vi "apply_deadband.vi"(10 "Deadband":dbl, 11 "Input":dbl) -> (3 "Input with deadband":dbl)   [LabVIEW 2012]
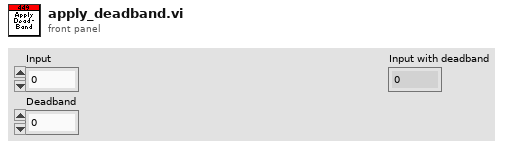
[diagram p1: front panel]
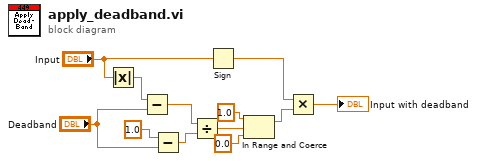
[diagram p0: block diagram]
diagram:
  n1 = Absolute Value(x="Input") -> (abs(x)=w12:dbl)
  n2 = Subtract(x=w12, y="Deadband") -> (x-y=w11:dbl)
  n3 = Subtract(x=1.0, y="Deadband") -> (x-y=w10:dbl)
  n4 = Divide(x=w11, y=w10) -> (x/y=w7:dbl)
  n5 = Sign(1:"Input") -> (0:w2:dbl)
  n6 = In Range and Coerce(upper limit=1.0 ("x"), x=w7, lower limit=0.0) -> (coerced(x)=w3:dbl)  [unwired: 1 out]
  n7 = Multiply(x=w2, y=w3) -> (x*y=→"Input with deadband":dbl)
